vi "RSZVB Window Close.vi"(8 "error in (no error)":errorcluster {"code" format="%.0x"}, 10 "Setup Name (Set1)":string="Set1", 11 "VISA session":refnum<visa-resource-name>) -> (0 "error out":errorcluster {"code" format="%.0x"}, 3 "dup VISA session":refnum<visa-resource-name>)   [LabVIEW 2011]
doc: "This VI closes the specified setup. If <Setup Name> is not specified (NULL), all existing setups are closed.\n\nRemote-control command(s):\nMEMory:DELete:ALL\nMEMory:DELete[:NAME] '<file_name>'"
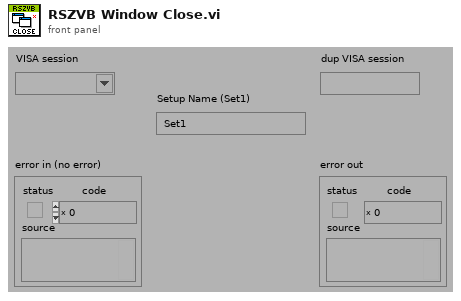
[diagram p1: front panel]
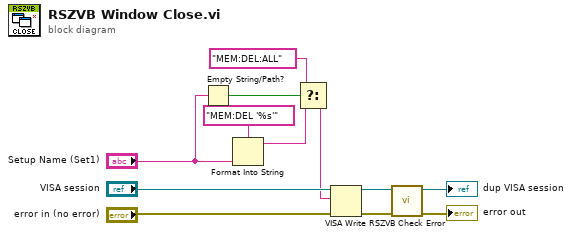
[diagram p0: block diagram]
diagram:
  n1 = Empty String/Path?(string/path="Setup Name (Set1)") -> (empty?=w4:bool)
  n2 = Format Into String(format string="MEM:DEL '%s'", "Setup Name (Set1)") -> (resulting string=w2:string)  [unwired: 2 in, 1 out]
  n3 = Select(t="MEM:DEL:ALL", s=w4, f=w2) -> (s? t:f=w3:string)
  n4 = VISA Write(VISA resource name="VISA session", write buffer=w3, error in (no error)="error in (no error)") -> (VISA resource name out=w12:refnum<visa-resource-name>, error out=w11:errorcluster)  [unwired: 1 out]
  n5 = call "RSZVB Check Error.vi"("error in (no error)"=w11, "VISA session"=w12) -> ("error out"=→"error out":errorcluster, "dup VISA session"=→"dup VISA session":refnum<visa-resource-name>)  [unwired: 8 in]
